vi "Find Insert Index for Offset.vi"(8 "error in (no error)":errorcluster, 10 "offset":u64, 11 "Transfer Configuration in":refnum<class "Configuration.Transfer.lvclass">) -> (0 "error out":errorcluster, 2 "index":i32, 3 "Transfer Configuration out":refnum<class "Configuration.Transfer.lvclass">)   [LabVIEW 2016, in "Data Sharing Framework.Configuration.lvlib" / "Configuration.Transfer.lvclass"]
uses:
  Configuration.Transfer.lvclass
  Configuration.Transfer.lvclass/Configuration.Transfer.ctl
  Configuration.Channel/Configuration.Channel.lvclass/Configuration.Channel.ctl
  Configuration.Channel/Configuration.Channel.lvclass
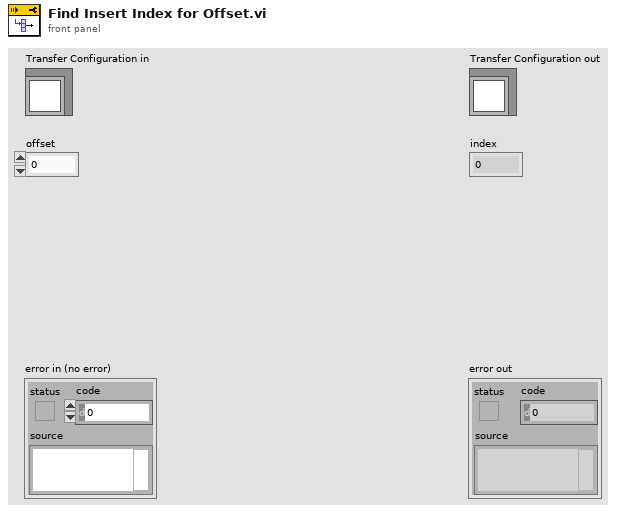
[diagram p1: front panel]
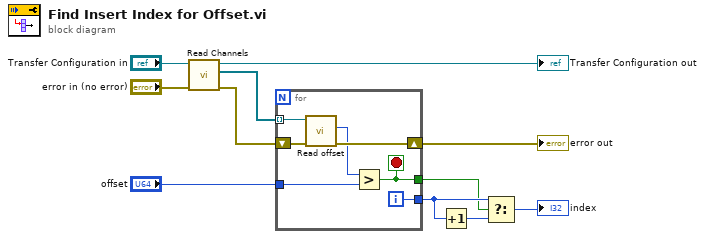
[diagram p0: block diagram]
diagram:
  n1 = call "Read Channels.vi"("error in (no error)"="error in (no error)", "Configuration.Transfer in"="Transfer Configuration in") -> ("error out"=w8:errorcluster, "Channels"=w10:refnum<class "Configuration.Channel.lvclass">[], "Configuration.Transfer out"=→"Transfer Configuration out":refnum<class "Configuration.Transfer.lvclass">)  [unwired: 7 in]
  n2 = for {
    tunnel: w10 -> [w18] mode=indexing
    tunnel: "offset" -> [w17]
    shift-right: [w15] -> w1
    shift-left: w8 -> [w16]
    tunnel: [w13] -> w3
    tunnel: [w12] -> w4
    i -> [w12]
    stop <- w13 stop-if-true
    n3 = call "Read offset.vi"("error in (no error)"=w16, "Configuration.Channel in"=w18) -> ("error out"=w15:errorcluster, "offset"=w14:u64)  [unwired: 7 in, 1 out]
    n4 = Greater?(x=w14, y=w17) -> (0:w13:bool)
  }
  "error out" <- w1
  n5 = Increment(x=w4) -> (x+1=w5:i32)
  n6 = Select(t=w4, s=w3, f=w5) -> (s? t:f=→"index":i32)
